vi "ReadSDO_FLT.vi"(4 "SubIndex":i32 format="%x", 6 "Index":i32 format="%x", 7 "nodeID":i32, 8 "error in (no error)":errorcluster, 9 "Instrument Ref In":refnum<k24>) -> (1 "SDO Float Result":sgl, 2 "error out":errorcluster, 3 "Instrument Ref Out":refnum<k24>)   [LabVIEW 2016]
uses:
  C:/user/patrick/hg/levylab_inst_ppms2/lvsrc/PPMS2/QDInstrument_LabView/QDInstrument.dll
  PPMS2/QDInstrument_LabView/QDInstrument.dll
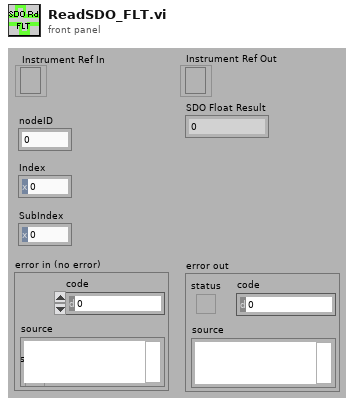
[diagram p1: front panel]
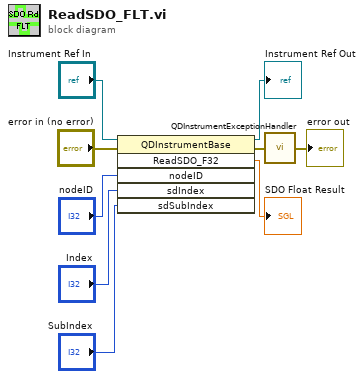
[diagram p0: block diagram]
diagram:
  n1 = invoke class="QDInstrumentBase" method="ReadSDO_F32"(reference="Instrument Ref In", error in="error in (no error)", "nodeID"="nodeID", "sdIndex"="Index", "sdSubIndex"="SubIndex") -> (reference out=→"Instrument Ref Out":refnum<k24>, error out=w2:errorcluster, "ReadSDO_F32"=→"SDO Float Result":sgl)  [unwired: 1 in, 3 out]
  n2 = call "QDInstrumentExceptionHandler.vi"("Error in"=w2) -> ("Error out"=→"error out":errorcluster)
